vi "merge_Timer Off Delay.vi"   [LabVIEW 2020, in "NI_FunctionBlockMergeVIs.lvlib"]
doc: "Generates an <B>output</B> signal with rising edges that align with the <B>input</B> signal, but with falling edges delayed by <B>preset time (ms)</B>."
uses:
  <vilib>/functionblocks/NI_FunctionBlockMergeVIs.lvlib
  <vilib>/functionblocks/FB Core/FB Core.xnode
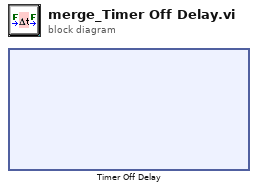
[diagram p0: block diagram]
diagram:
  n1 = xnode "Timer Off Delay"() -> ()  [unwired: 3 in, 3 out]
